vi "ZMC Get Sys Specification.vi"(8 "error in (no error)":errorcluster caption="错误输入（无错误）", 10 "pspeci":T1, 11 "handle":u32) -> (0 "error out":errorcluster caption="错误输出", 1 "function return":i32, 2 "pspeci out":T1, 3 "handle out":u32)   [LabVIEW 2015, in "zauxdll.lvlib"]
doc: "int32 __stdcall ZMC_GetSysSpecification(ZMC_HANDLE handle, struct_SysMaxSpecification *pspeci);"
uses:
  zauxdll.lvlib
  zmotion.dll
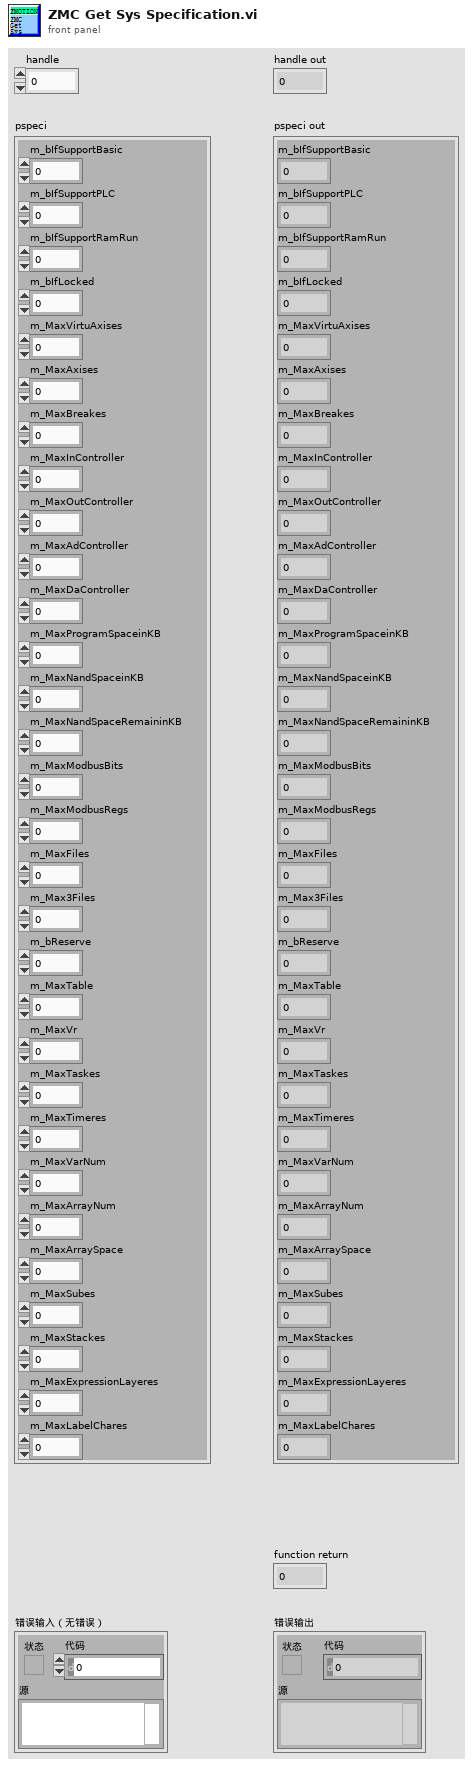
[diagram p1: front panel]
types:
  T1 = cluster{"m_bIfSupportBasic":u8, "m_bIfSupportPLC":u8, "m_bIfSupportRamRun":u8, "m_bIfLocked":u8, "m_MaxVirtuAxises":u16, "m_MaxAxises":u8, "m_MaxBreakes":u8, "m_MaxInController":u8, "m_MaxOutController":u8, "m_MaxAdController":u8, "m_MaxDaController":u8, "m_MaxProgramSpaceinKB":u32, "m_MaxNandSpaceinKB":u32, "m_MaxNandSpaceRemaininKB":u32, "m_MaxModbusBits":u16, "m_MaxModbusRegs":u16, "m_MaxFiles":u16, "m_Max3Files":u8, "m_bReserve":u8, "m_MaxTable":u32, "m_MaxVr":u32, "m_MaxTaskes":u16, "m_MaxTimeres":u16, "m_MaxVarNum":u16, "m_MaxArrayNum":u16, "m_MaxArraySpace":u32, "m_MaxSubes":u16, "m_MaxStackes":u16, "m_MaxExpressionLayeres":u16, "m_MaxLabelChares":u16}
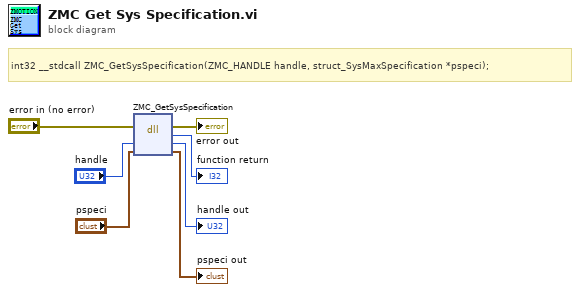
[diagram p0: block diagram]
diagram:
  # "int32 __stdcall ZMC_GetSysSpecification(ZMC_HANDLE handle, struct_SysMaxSpecification *pspeci);"
  n1 = dll-call lib="C:/Users/VIC/Desktop/GOGORO_SA/system/LLB/zmotion/zaux/zmotion.*" fn="ZMC_GetSysSpecification"(error in="error in (no error)", "handle"="handle", "pspeci"="pspeci") -> (error out=→"error out":errorcluster, →"function return":i32, "handle"=→"handle out":u32, "pspeci"=→"pspeci out":T1)  [unwired: 2 in, 1 out]
